vi "SW_Shape_Conditions_Array_after_Loading_XML.vi"(2 "error in (no error)":errorcluster, 3 "Condition presets loaded in":T1) -> (0 "error out":errorcluster, 1 "Conditions presets array out":T2 {"Specifier(s)"."Validity criteria(s)"."Validity value" min=0.0 step=0.1 format="%.2g"; "Specifier(s)"."Value" step=1.0 format="%#.2g"})   [LabVIEW 2018, in "Tracker.lvlib"]
uses:
  Tracker.lvlib
  Controls/CTL_Conditions_Array.ctl
  Controls/CTL_Conditions_Cluster.ctl
  Controls/CTL_Condition_type.ctl
  Controls/CTL_Comparison_type.ctl
  Controls/CTL_Validity_check_criteria.ctl
  Controls/CTL_Response_info.ctl
  Controls/CTL_Condition_response_type.ctl
  Controls/CTL_Reponse_port_info.ctl
  Controls/CTL_Conditions_All_Presets_Cluster.ctl
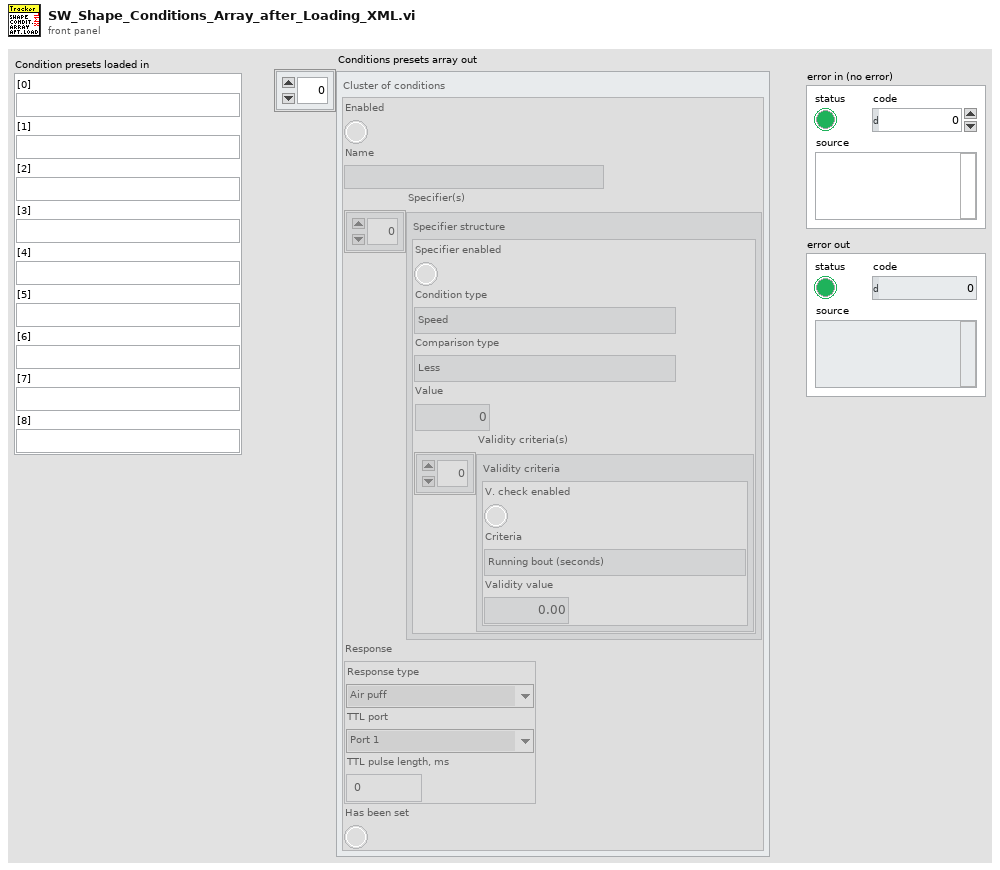
[diagram p1: front panel]
types:
  T1 = typedef "Tracker.lvlib/CTL_Conditions_All_Presets_Cluster.ctl" = cluster{"[0]":string, "[1]":string, "[2]":string, "[3]":string, "[4]":string, "[5]":string, "[6]":string, "[7]":string, "[8]":string}
  T2 = typedef "Tracker.lvlib/CTL_Conditions_Array.ctl" = T3[]
  T3 = typedef "Tracker.lvlib/CTL_Conditions_Cluster.ctl" = cluster{"Enabled":bool, "Name":string, "Specifier(s)":cluster{"Specifier enabled":bool, "Condition type":T4, "Comparison type":T5, "Value":dbl, "Validity criteria(s)":cluster{"V. check enabled":bool, "Criteria":T6, "Validity value":dbl}[]}[], "Response":T7, "Has been set":bool}
  T4 = typedef "Tracker.lvlib/CTL_Condition_type.ctl" = enum16{"Speed", "Zone", "Angle to wall"}
  T5 = typedef "Tracker.lvlib/CTL_Comparison_type.ctl" = enum16{"Less", "Less or Equal", "Equal", "Greater or Equal", "Greater", "Not Equal"}
  T6 = typedef "Tracker.lvlib/CTL_Validity_check_criteria.ctl" = enum16{"Running bout (seconds)", "Running bout (meters)"}
  T7 = typedef "Tracker.lvlib/CTL_Response_info.ctl" = cluster{"Response type":T8, "TTL port":T9, "TTL pulse length, ms":dbl}
  T8 = typedef "Tracker.lvlib/CTL_Condition_response_type.ctl" = enum16{"None", "Air puff", "Liquid reward"}
  T9 = typedef "Tracker.lvlib/CTL_Reponse_port_info.ctl" = enum16{"Port 1", "Port 2", "Port 3", "Port 4"}
  T10 = cluster{"Boolean Round":bool, "code":i32, "source":string}
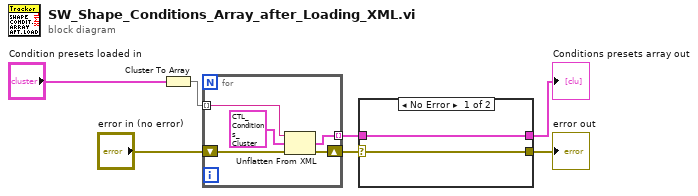
[diagram p0: block diagram]
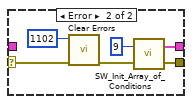
[diagram p2: hidden frame]
diagram:
  n1 = Cluster To Array(cluster="Condition presets loaded in") -> (array=w3:string[])
  n2 = for {
    tunnel: w3 -> [w8] mode=indexing
    tunnel: [w11] -> w2 mode=indexing
    shift-right: [w9] -> w1
    shift-left: "error in (no error)" -> [w10]
    n3 = Unflatten From XML(xml string=w8, type=T3 {"Enabled"=FALSE, "Name"="", "Specifier(s)"=[], "Response"={"Response type"=enum."Air puff", "TTL port"=enum."Port 1", "TTL pulse length, ms"=0.0}, "Has been set"=FALSE} ("Cluster of conditions"), error in (no error)=w10) -> (value=w11:T3, error out=w9:errorcluster)
  }
  n4 = case shown="No Error" w1 {
    selector: w1 -> [w14 w18]
    tunnel: [w14 w16] -> w7
    tunnel: [w13 w19] -> w6
    tunnel: w2 -> [w13 _]
    frame No Error {
    }
    frame Error {
      n5 = call <vilib>:"Clear Errors.vi"("error in (no error)"=w18, "specific error code to clear (0: all)"=1102) -> ("error out"=w17:errorcluster)  [unwired: 4 in, 1 out]
      n6 = call "SW_Init_Array_of_Conditions.vi"("error in (no error)"=w17, "Array size"=9) -> ("error out"=w16:T10, "Array of conditions"=w19:T2)
    }
  }
  "Conditions presets array out" <- w6
  "error out" <- w7
